vi "UpDown Counter.vi"() -> ()   [LabVIEW 2025]
doc: "This example uses two digital lines to count up and down. TTL pulses on one digital channel increase the count, while TTL pulses on the other digital channel decrease the count.\n\nThis example expects a USB cable connected from your development PC to the Type B USB Jack (next to the power input) on the roboRIO.\n\nThis example expects the Driver Station to be running."
uses:
  <vilib>/Rock Robotics/SystemInterfaces/DIO/FPGA_DIOChannel.ctl
  <vilib>/Rock Robotics/WPI/Counter/WPI_CounterDigitalInputToDigitalSource.vi
  <vilib>/Rock Robotics/WPI/Counter/WPI_CounterOpen UpDown Mode.vi
panel:
  in  "Number of Period Samples to Average":u8=1 min=1 max=128
  in  "UpEdge":T1(ring)
  in  "DownEdge":T1(ring)
  in  "Counter Down Channel":T2=enum."DIO 8"
  out "Counter Status":string
  in  "Counter Up Channel":T2=enum."DIO 7"
  in  "Maximum Period (sec)":dbl=5.0
  in  "Counter Reset":bool
  in  "Stop":bool
  out "Counter Value":i32
  out "Period (sec)":dbl
  # "Set these inputs before running."
  # "This can be set while running."
  # "Counter Output Information"
  # "Signal\nUpEdge ------\nDownEdge ---"
  # "roboRIO\nDIO-7  S\nDIO-8  S"
  # "TTL Signals"
  # "This shows wiring for TTL signals."
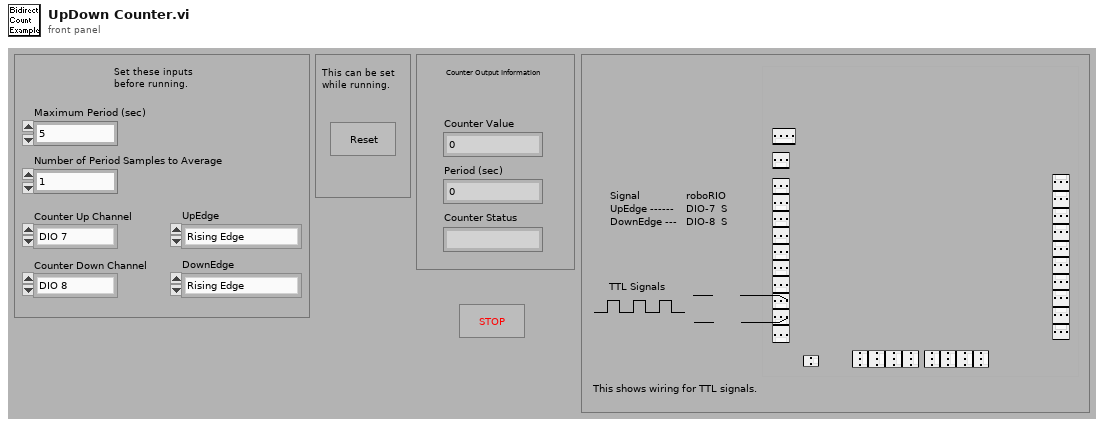
[diagram p1: front panel]
types:
  T1 = enum16{"Rising Edge", "Falling Edge", "Raising & Falling Edge", "Disabled"}
  T2 = typedef "FPGA_DIOChannel.ctl" = enum8{"DIO 0", "DIO 1", "DIO 2", "DIO 3", "DIO 4", "DIO 5", "DIO 6", "DIO 7", "DIO 8", "DIO 9", "DIO MXP 0", "DIO MXP 1", "DIO MXP 2", "DIO MXP 3", "DIO MXP 4", "DIO MXP 5", "DIO MXP 6", "DIO MXP 7", "DIO MXP 8", "DIO MXP 9", "DIO MXP 10", "DIO MXP 11", "DIO MXP 12", "DIO MXP 13", "DIO MXP 14", "DIO MXP 15", "SPI Port CS1", "SPI Port CS2", "SPI Port CS3", "SPI Port MISO", "SPI Port MOSI", "Invalid"}
  T3 = typedef "WPI_DigitalInputDevRef.ctl" = cluster{"DevStatus":errorcluster, "DIO Channel":T2}
  T4 = typedef "FPGA_CounterEncoderSourceConvertionLVSourceType.ctl" = cluster{"DevStatus":errorcluster, "AnalogTriggerMode?":bool, "DigitalMode":cluster{"DIO Channel":T5}, "AnalogTriggerMode":cluster{"AnalogTriggerIndex":T6, "OutputType":T7}}
  T5 = typedef "FPGA_DIODigitalSourceChannel.ctl" = enum8{"DIO 0", "DIO 1", "DIO 2", "DIO 3", "DIO 4", "DIO 5", "DIO 6", "DIO 7", "DIO 8", "DIO 9", "DIO MXP 0", "DIO MXP 1", "DIO MXP 2", "DIO MXP 3", "DIO MXP 4", "DIO MXP 5", "DIO MXP 6", "DIO MXP 7", "DIO MXP 8", "DIO MXP 9", "DIO MXP 10", "DIO MXP 11", "DIO MXP 12", "DIO MXP 13", "DIO MXP 14", "DIO MXP 15", "SPI Port CS1", "SPI Port CS2", "SPI Port CS3", "SPI Port MISO", "SPI Port MOSI", "Disabled"}
  T6 = typedef "FPGA_AnalogTriggerIndex.ctl" = enum8{"Trig 0", "Trig 1", "Trig 2", "Trig 3", "Trig 4", "Trig 5", "Trig 6", "Trig 7", "Invalid"}
  T7 = typedef "FPGA_AnalogTriggerOutType.ctl" = enum16{"InWindow", "TriggerState", "Rising", "Falling"}
  T8 = typedef "WPI_CounterDevRef.ctl" = cluster{"DevStatus":errorcluster, "CntIndex":T9}
  T9 = typedef "FPGA_CounterCtrSystemIndex.ctl" = enum8{"Ctr 0", "Ctr 1", "Ctr 2", "Ctr 3", "Ctr 4", "Ctr 5", "Ctr 6", "Ctr 7", "Invalid"}
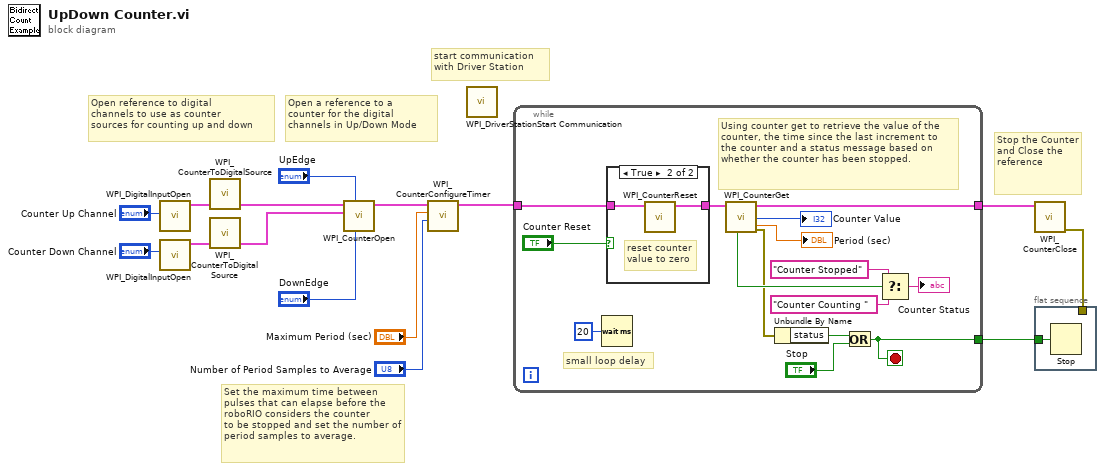
[diagram p0: block diagram]
diagram:
  # "start communication with Driver Station"
  # "Stop the Counter and Close the reference"
  # "Open a reference to a\ncounter for the digital \nchannels in Up/Down Mode"
  # "Set the maximum time between pulses that can elapse before the roboRIO considers the counter \nto be stopped and set the number of period samples to average."
  # "Open reference to digital \nchannels to use as counter\nsources for counting up and down"
  n1 = call <vilib>:"WPI_DigitalInputOpen.vi"("DIO Channel"="Counter Up Channel") -> ("DigitalInputDevRef"=w13:T3)  [unwired: 1 in, 9 out]
  n2 = call <vilib>:"WPI_DigitalInputOpen.vi"("DIO Channel"="Counter Down Channel") -> ("DigitalInputDevRef"=w11:T3)  [unwired: 1 in, 9 out]
  n3 = call-poly <vilib>:"WPI_CounterToDigitalSource.vi"("DigitalInputDevRef"=w13) -> ("Digital Source"=w15:T4)  [unwired: 6 out]
  n4 = call-poly <vilib>:"WPI_CounterToDigitalSource.vi"("DigitalInputDevRef"=w11) -> ("Digital Source"=w10:T4)  [unwired: 6 out]
  n5 = call-poly <vilib>:"WPI_CounterOpen.vi"("DownEdge"="DownEdge", "UpEdge"="UpEdge", "Down Source"=w10, "Up Source"=w15) -> ("CounterDevRef"=w8:T8)  [unwired: 3 in, 4 out]
  n6 = call <vilib>:"WPI_CounterConfigureTimer.vi"("Number Samples to Average"="Number of Period Samples to Average", "MaxPeriod (sec)"="Maximum Period (sec)", "CounterDevRef in"=w8) -> ("CounterDevRef out"=w2:T8)  [unwired: 1 in, 7 out]
  n7 = call <vilib>:"WPI_DriverStationStart Communication.vi"() -> ()  [unwired: 3 in, 9 out]
  n8 = while {
    tunnel: [w28] -> w1
    tunnel: w2 -> [w26]
    tunnel: [w18] -> w4
    stop <- w18 stop-if-true
    # "small loop delay"
    # "Using counter get to retrieve the value of the counter, the time since the last increment to the counter and a status message based on whether the counter has been stopped."
    n9 = Wait (ms)(milliseconds to wait=u32 20) -> ()  [unwired: 1 out]
    n10 = case shown="True" "Counter Reset" {
      tunnel: w26 -> [w31 w33]
      tunnel: [w31 w32] -> w25
      frame False {
      }
      frame True {
        # "reset counter value to zero"
        n11 = call <vilib>:"WPI_CounterReset.vi"("CounterDevRef in"=w33) -> ("CounterDevRef out"=w32:T8)  [unwired: 1 in, 9 out]
      }
    }
    n12 = call <vilib>:"WPI_CounterGet.vi"("CounterDevRef in"=w25) -> ("error out"=w21:errorcluster, "Value"=→"Counter Value":i32, "CounterDevRef out"=w28:T8, "Period (sec)"=→"Period (sec)":dbl, "Stopped"=w24:bool)  [unwired: 1 in, 5 out]
    n13 = Unbundle By Name(w21) -> ("status"=w20:bool)
    n14 = Or(x=w20, y="Stop") -> (x .or. y?=w18:bool)
    n15 = Select(t="Counter Stopped", s=w24, f="Counter Counting ") -> (s? t:f=→"Counter Status":string)
  }
  n16 = call <vilib>:"WPI_CounterClose.vi"("CounterDevRef"=w1) -> ("error out"=w3:errorcluster)  [unwired: 2 in, 8 out]
  n17 = flat-sequence {
    tunnel: w4 -> [w34]
    tunnel: w3 -> [_]
    frame #0 {
      n18 = Stop(stop? (T)=w34) -> ()
    }
  }
